vi "Arduino_Read_PWM_Voltage_Array.vi"(8 "error in (no error)":errorcluster, 11 "Connection In":refnum<k5>) -> (0 "error out":errorcluster, 2 "Output Array":dbl[](array[numeric]), 3 "Connection Out":refnum<k5>)   [LabVIEW 2020]
panel:
  out "write":u32
  out "read":u32
  # "TIME TAKEN"
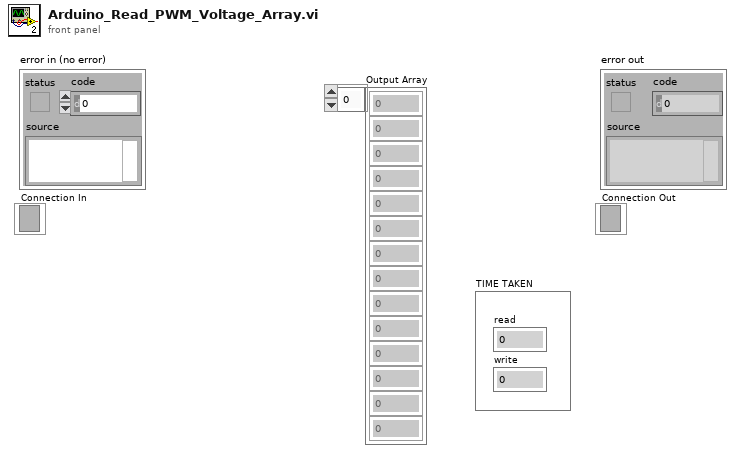
[diagram p1: front panel]
types:
  T1 = enum16{"Standard", "Buffered", "CRLF", "Immediate"}
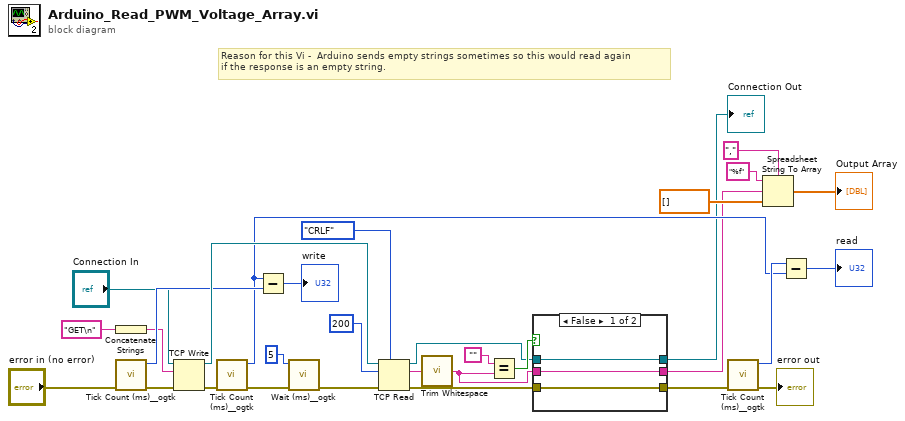
[diagram p0: block diagram]
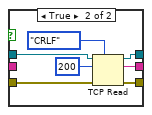
[diagram p2: hidden frame]
diagram:
  # "Reason for this Vi -  Arduino sends empty strings sometimes so this would read again\nif the response is an empty string."
  n1 = Concatenate Strings("GET\n" ("data in")) -> (w16:string)
  n2 = call "Tick Count (ms)__ogtk.vi"("error in (no error)"="error in (no error)") -> ("error out"=w24:errorcluster, "millisecond timer value"=w22:u32)  [unwired: 9 in]
  n3 = TCP Write(connection ID="Connection In", data in=w16, error in (no error)=w24) -> (connection ID out=w31:refnum<k5>, error out=w23:errorcluster)  [unwired: 1 in, 1 out]
  n4 = call "Tick Count (ms)__ogtk.vi"("error in (no error)"=w23) -> ("error out"=w15:errorcluster, "millisecond timer value"=w20:u32)  [unwired: 9 in]
  n5 = Subtract(x=w20, y=w22) -> (x-y=→"write":u32)
  n6 = call "Wait (ms)__ogtk.vi"("error in (no error)"=w15, "milliseconds to wait"=u32 5) -> ("error out"=w14:errorcluster)  [unwired: 8 in, 1 out]
  n7 = TCP Read(connection ID=w31, bytes to read=200, error in (no error)=w14, 7:T1."CRLF" ("mode (standard)")) -> (connection ID out=w9:refnum<k5>, data out=w12:string, error out=w8:errorcluster)  [unwired: 1 in]
  n8 = call "Trim Whitespace.vi"("string"=w12) -> ("trimmed string"=w5:string)  [unwired: 1 in]
  n9 = Equal?(x="", y=w5) -> (x = y?=w10:bool)
  n10 = case shown="False" w10 {
    tunnel: w9 -> [w32 w39]
    tunnel: [w32 w38] -> w1
    tunnel: w8 -> [w33 w37]
    tunnel: [w33 w36] -> w7
    tunnel: [w34 w35] -> w6
    tunnel: w5 -> [w34 _]
    frame False {
    }
    frame True {
      n11 = TCP Read(connection ID=w39, bytes to read=200, error in (no error)=w37, 7:T1."CRLF" ("mode (standard)")) -> (connection ID out=w38:refnum<k5>, data out=w35:string, error out=w36:errorcluster)  [unwired: 1 in]
    }
  }
  "Connection Out" <- w1
  n12 = call "Tick Count (ms)__ogtk.vi"("error in (no error)"=w7) -> ("error out"=→"error out":errorcluster, "millisecond timer value"=w21:u32)  [unwired: 9 in]
  n13 = Spreadsheet String To Array(delimiter (Tab)=",", format string="%f", spreadsheet string=w6, array type (2D Dbl)=dbl[] []) -> (array=→"Output Array":dbl[])
  n14 = Subtract(x=w21, y=w20) -> (x-y=→"read":u32)
